vi "SM-s_Timed Loop Error & Abort.vi"(8 "Error - State In":errorcluster, 9 "Timed Loop Error In":errorcluster, 11 "Wakeup Reason":T1) -> (0 "error out":errorcluster)   [LabVIEW 2018]
doc: "Combines the Error clusters of a Timed Loop left internal node Error with the Error from an external State Machine Shift Variable and also checks for a Timed Loop Wakeup Reason of \"Aborted\".\n\nIF Aborted THEN Error Out is TRUE, Code is -9999 and source is \"Aborted\". This lets the State Machine control select the Exit or Aborted case for the final iteration of the Timed Loop.\n\n2007_12_27 Mike Ashe\nmichael.ashe@imaginatics.net\nCell: 860-961-0876"
uses:
  <vilib>/Platform/TimedLoop/XDataNode/wakeup.ctl
  <vilib>/Platform/TimedLoop/XDataNode/XDNodeRunTimeDep.lvlib
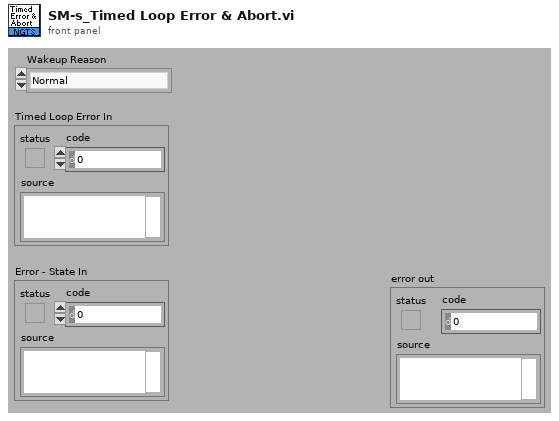
[diagram p1: front panel]
types:
  T1 = typedef "XDNodeRunTimeDep.lvlib/wakeup.ctl" = enum32{"Normal", "Aborted", "Asynchronous wakeup", "Timing source error", "Timed loop error", "Timeout"}
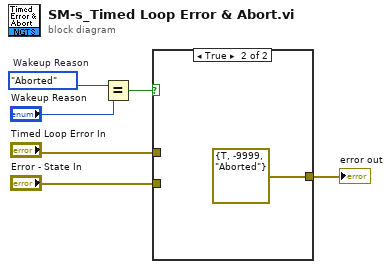
[diagram p0: block diagram]
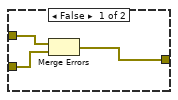
[diagram p2: hidden frame]
diagram:
  w4 = wakeup."Aborted"  # Wakeup Reason
  n1 = Equal?(x=w4, y="Wakeup Reason") -> (x = y?=w3:bool)
  n2 = case shown="True" w3 {
    tunnel: [w9 errorcluster {"status"=TRUE, "code"=-9999, "source"="Aborted"} ("error out")] -> w6
    tunnel: "Error - State In" -> [w8 _]
    tunnel: "Timed Loop Error In" -> [w7 _]
    frame False {
      n3 = Merge Errors(w7, w8) -> (w9:errorcluster)
    }
    frame True {
    }
  }
  "error out" <- w6
